vi "Configure Timer Parameters.vi"(0 "VISA resource name":refnum<visa-resource-name>, 1 "Unit Address (1)":u8=1 min=1 max=254, 5 "Timer Start Threshold (0)":sgl min=0 max=9999, 9 "Timer Resolution Units (0)":u8(ring) items=["Per Hour", "Per Minute"], 11 "error in (no error)":errorcluster, 12 "Timer End Type (1)":u16(ring)=1 items=["Off", "Dwell", "SP2", "Reset"]) -> (4 "VISA resource name out":refnum<visa-resource-name>, 15 "error out":errorcluster)   [LabVIEW 2010, in "Eurotherm 32xx Series.lvlib"]
doc: "This VI sets Programmer/Timer parameters."
uses:
  <instrlib>/Eurotherm 32xx Series/Eurotherm 32xx Series.lvlib
panel:
  # "DWELL"
  # "SP2"
  # "OFF"
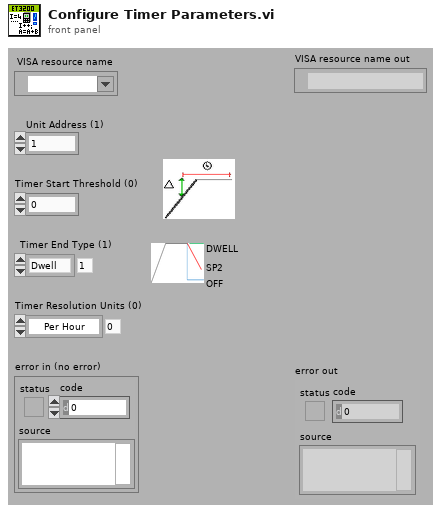
[diagram p1: front panel]
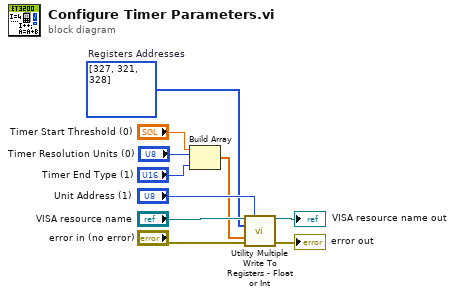
[diagram p0: block diagram]
diagram:
  w4 = u16[] [327, 321, 328]  # Registers Addresses
  n1 = Build Array("Timer Start Threshold (0)", "Timer Resolution Units (0)", "Timer End Type (1)") -> (w5:sgl[])
  n2 = call <instrlib>:"Utility Multiple Write To Registers - Float or Int.vi"("VISA resource name"="VISA resource name", "Unit Address (1)"="Unit Address (1)", "Registers Addresses (0)"=w4, "Data (0)"=w5, "error in (no error)"="error in (no error)") -> ("VISA resource name out"=→"VISA resource name out":refnum<visa-resource-name>, "error out"=→"error out":errorcluster)  [unwired: 9 in]
